vi "Read Process.vi"(11 "CommonState in":refnum<class "CoordinatorState.lvclass">) -> (2 "Process Enqueuer":refnum<class "Message Enqueuer.lvclass">, 3 "CommonState out":refnum<class "CoordinatorState.lvclass">)   [LabVIEW 2014, in "States.lvlib" / "CoordinatorState.lvclass"]
doc: "Returns the enqueuer for the nested Process Actor."
uses:
  CoordinatorState.lvclass
  <vilib>/ActorFramework/Message Enqueuer/Message Enqueuer.lvclass
  CoordinatorState.lvclass/CoordinatorState.ctl
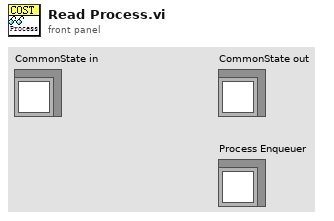
[diagram p1: front panel]
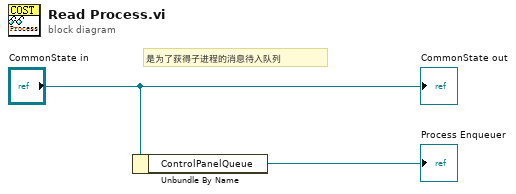
[diagram p0: block diagram]
diagram:
  # "是为了获得子进程的消息待入队列"
  n1 = Unbundle By Name("CommonState in") -> ("ControlPanelQueue"=→"Process Enqueuer":refnum<class "Message Enqueuer.lvclass">)
  "CommonState out" <- "CommonState in"
